vi "instrumentProperties_PDTemperatureMode_available.vi"(0 "reference":refnum<class "OSA200.lvclass">, 5 "error in (no error)":errorcluster) -> (14 "duplicate reference":refnum<class "OSA200.lvclass">, 16 "PDTempCtrl_available":bool, 19 "error out":errorcluster)   [LabVIEW 2010, in "OSA200.lvclass"]
doc: "Returns boolean true if the active channel photodetector, (channel assigned for acquisition), is held at constant low temperature, (cooled).\n\nNote - OSA200 series has only one channel."
uses:
  OSA200.lvclass
  OSA.lvclass
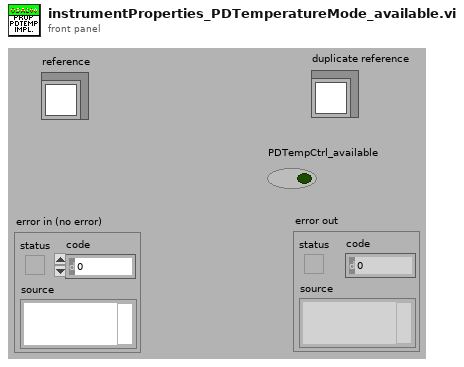
[diagram p1: front panel]
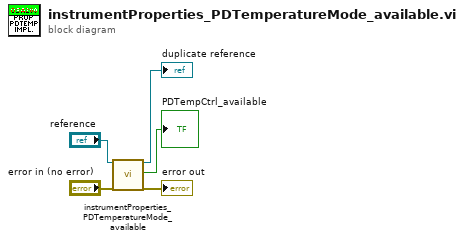
[diagram p0: block diagram]
diagram:
  n1 = call-parent "instrumentProperties_PDTemperatureMode_available.vi"("reference"="reference", "error in (no error)"="error in (no error)") -> ("duplicate reference"=→"duplicate reference":refnum<class "OSA200.lvclass">, "PDTempCtrl_available"=→"PDTempCtrl_available":bool, "error out"=→"error out":errorcluster)  [unwired: 15 in]
